vi "Get Meta Data (UDP).vi"(8 "error in":errorcluster, 11 "connection info in":T1) -> (0 "error out":errorcluster, 3 "connection info out":T1, 5 "meta data":T2[](array[typedef]))   [LabVIEW 2013, in "NI STM.lvlib"]
doc: "Returns the meta data associated with the STM session."
uses:
  NI STM.lvlib
  UDP Connection Info.ctl
  SubVIs/MetaDataElement.ctl
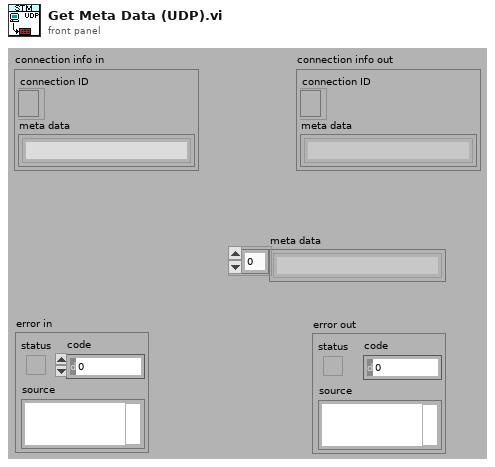
[diagram p1: front panel]
types:
  T1 = typedef "NI STM.lvlib/UDP Connection Info.ctl" = cluster{"connection ID":refnum<k16>, "meta data":T2[]}
  T2 = typedef "NI STM.lvlib/MetaDataElement.ctl" = string
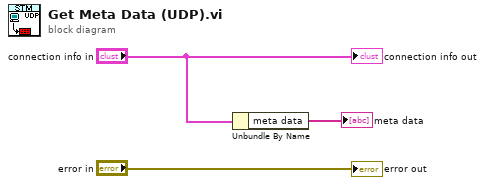
[diagram p0: block diagram]
diagram:
  n1 = Unbundle By Name("connection info in") -> ("meta data"=→"meta data":T2[])
  "connection info out" <- "connection info in"
  "error out" <- "error in"
